vi "ma_Check Segmented Limit (single segment formula).vi"(0 "Specification Cluster":cluster{"X":dbl[], "Y":string[]} {"X" format="%0.2f"}, 1 "x0":dbl format="%0.2f", 2 "dx":dbl format="%0.2f", 3 "error in":errorcluster) -> (8 "limit spec ok":bool, 10 "error out":errorcluster)   [LabVIEW 2020, in "NI_MAPro.lvlib"]
uses:
  NI_MAPro.lvlib
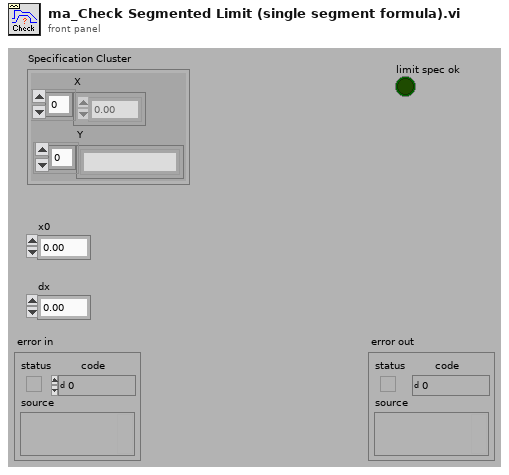
[diagram p1: front panel]
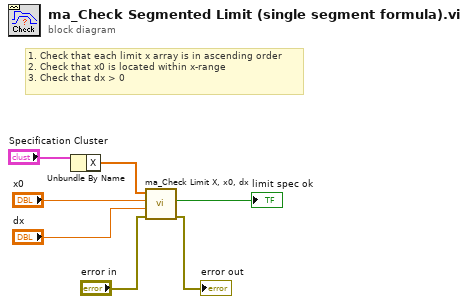
[diagram p0: block diagram]
diagram:
  # "1. Check that each limit x array is in ascending order\n2. Check that x0 is located within x-range\n3. Check that dx > 0"
  n1 = Unbundle By Name("Specification Cluster") -> ("X"=w2:dbl[])
  n2 = call "ma_Check Limit X, x0, dx.vi"("X"=w2, "x0"="x0", "dx"="dx", "error in"="error in") -> ("limit spec ok"=→"limit spec ok":bool, "error out"=→"error out":errorcluster)  [unwired: 5 out]
